vi "실습2-2여러숫자더하기.vi"() -> ()   [LabVIEW 2014]
panel:
  out "A 7":dbl
  in  "A 6":dbl
  in  "A 5":dbl
  in  "A 4":dbl
  in  "A 3":dbl
  in  "A 2":dbl
  in  "A":dbl
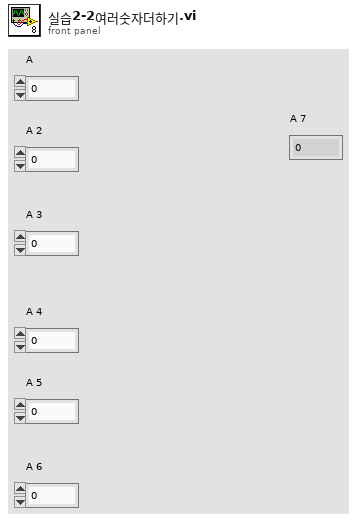
[diagram p1: front panel]
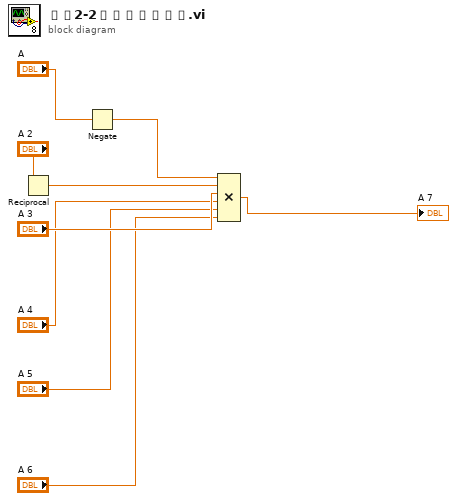
[diagram p0: block diagram]
diagram:
  n1 = Reciprocal(x="A 2") -> (1/x=w2:dbl)
  n2 = Negate(x="A") -> (-x=w1:dbl)
  n3 = Compound Arithmetic op=MULTIPLY(w1, w2, "A 3", "A 4", "A 5", "A 6") -> (→"A 7":dbl)
